vi "location_y.vi"() -> ()   [LabVIEW 2018]
panel:
  in  "当前位置-Y":dbl
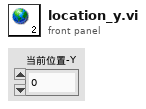
[diagram p1: front panel]
diagram:
